vi "Model Cleanup Done.vi"(11 "IModel in":refnum<class "IModel.lvclass">) -> (3 "IModel out":refnum<class "IModel.lvclass">)   [LabVIEW 2020, in "IModel.lvlib" / "IModel.lvclass"]
uses:
  <vilib>/gpm_packages/@cs/mva-core/Source/IModel/IModel/IModel.lvclass
  C:/Program Files/National Instruments/LabVIEW 2020/vi.lib/ActorFramework/Actor/Actor.lvclass
  C:/Program Files/National Instruments/LabVIEW 2020/vi.lib/gpm_packages/@cs/mva-core/Source/IObserver/IObserver/IObserver.lvclass
  <vilib>/ActorFramework/Actor/Actor.lvclass/Actor.ctl
  <vilib>/ActorFramework/Message Enqueuer/Message Enqueuer.lvclass/Message Enqueuer.ctl
  <vilib>/gpm_packages/@cs/mva-core/Source/IModel/IModel/IModel.lvclass/IModel.ctl
  <vilib>/ActorFramework/Message/Message.lvclass
  <vilib>/gpm_packages/@cs/mva-core/Source/IObserver/IObserver/IObserver.lvclass/IObserver.ctl
  <vilib>/gpm_packages/@cs/event-logger/Source/Composed Log/LoggerReference/LoggerReference.lvclass/LoggerReference.ctl
  <vilib>/ActorFramework/Message Enqueuer/Init from Existing Queue.vi
  <vilib>/gpm_packages/@cs/event-logger/Source/Composed Log/LoggerReference/Log Event.vi
  <vilib>/gpm_packages/@cs/event-logger/Source/Composed Log/LoggerReference/Log.vi
  <vilib>/gpm_packages/@cs/event-logger/Source/Composed Log/LoggerReference/Get Valid Event Time.vi
  <vilib>/gpm_packages/@cs/event-logger/Source/Composed Log/LoggerReference/Remove Stale Logs.vi
  <vilib>/ActorFramework/Message Priority Queue/Priority Enqueue.vi
  <vilib>/Utility/LVClass/Get LV Class Name.vi
  <vilib>/ActorFramework/Message Enqueuer/Message Enqueuer.lvclass
  <vilib>/ActorFramework/Actor/Actor.lvclass
  <vilib>/gpm_packages/@cs/mva-core/Source/IObserver/IObserver/IObserver.lvclass
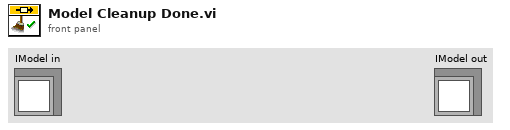
[diagram p1: front panel]
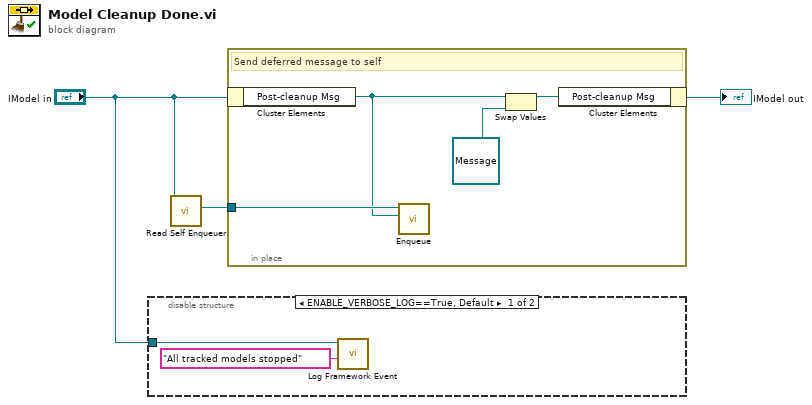
[diagram p0: block diagram]
diagram:
  n1 = disable-structure shown="ENABLE_VERBOSE_LOG==True, Default" {
    disable-tunnel: "IModel in" -> [w4 _]
    frame condition #0 (active) {
      # "Log end-of-shutdown event"
      n2 = call <vilib>:"Log Framework Event.vi"("Data To Log"="All tracked models stopped" ("Description"), "IObserver in"=w4) -> ()  [unwired: 9 in, 1 out]
    }
    frame condition #1 {
      # "Remove logging at compile time"
    }
  }
  n3 = call <vilib>:"Read Self Enqueuer.vi"("Actor"="IModel in") -> ("Self Enqueuer"=w3:refnum<class "Message Enqueuer.lvclass">)  [unwired: 10 in]
  n4 = in-place {
    in-place-border: w3 -> [w9]
    # "Send deferred message to self"
    n5 = in-place-cluster #1("IModel in") -> ("Post-cleanup Msg"=w8:refnum<class "Message.lvclass">)
    n6 = call <vilib>:"Enqueue.vi"("Message"=w8, "Message Enqueuer in"=w9) -> ()  [unwired: 8 in, 2 out]
    n7 = Swap Values(12:w8, 14:refnum<class "Message.lvclass"> refnum ("Final Last Ack Message")) -> (1:w7:refnum<class "Message.lvclass">)  [unwired: 1 in, 1 out]
    n8 = in-place-cluster #1("Post-cleanup Msg"=w7) -> (→"IModel out":refnum<class "IModel.lvclass">)
  }
